vi "Read Imagedata single Trial.vi"(5 "max value":dbl, 6 "Channel":i32=1, 8 "Experiment Parameters":T1, 9 "Current Plane":i32, 10 "Trial Number":i32, 11 "TDMS references(All Trials)":refnum<k34>[](array[refnum])) -> (3 "Image Array(Single Trial)":u8[][][](array[numeric]))   [LabVIEW 2017]
uses:
  Typedefs/Experiment Parameters.ctl
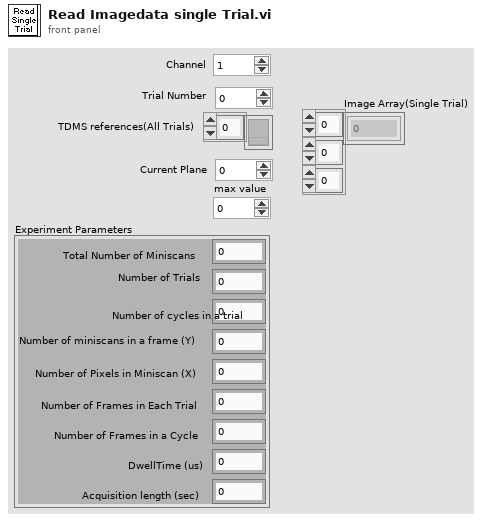
[diagram p1: front panel]
types:
  T1 = typedef "Experiment Parameters.ctl" = cluster{"Total Number of Miniscans":i32, "Number of Trials":i32, "Number of cycles in a trial":i32, "Number of miniscans in a frame (Y)":i32, "Number of Pixels in Miniscan (X)":i32, "Number of Frames in Each Trial":i32, "Number of Frames in a Cycle":i32, "DwellTime (us)":dbl, "Acquisition length (sec)":dbl}
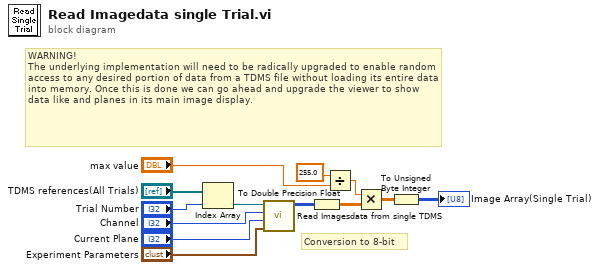
[diagram p0: block diagram]
diagram:
  # "Conversion to 8-bit"
  # "WARNING!\nThe underlying implementation will need to be radically upgraded to enable random access to any desired portion of data from a TDMS file without loading its entire data into memory. Once this is done we can go ahead and upgrade the viewer to show data like and planes in its main image display."
  n1 = Index Array(array="TDMS references(All Trials)", index="Trial Number") -> (element=w10:refnum<k34>)
  n2 = call "Read Imagesdata from single TDMS.vi"("Experiment Parameters"="Experiment Parameters", "Current Plane"="Current Plane", "Channel"="Channel", "Current Trial TDMS Ref"=w10) -> ("Image Array"=w2:i16[][][])  [unwired: 6 in, 1 out]
  n3 = To Double Precision Float(number=w2) -> (double precision float=w3:dbl[][][])
  n4 = Divide(x=255.0 ("Numeric"), y="max value") -> (x/y=w6:dbl)
  n5 = Multiply(x=w6, y=w3) -> (x*y=w5:dbl[][][])
  n6 = To Unsigned Byte Integer(number=w5) -> (unsigned 8bit integer=→"Image Array(Single Trial)":u8[][][])
